vi "ABB Norma 5000 panel.vi"() -> ()   [LabVIEW 2017]
uses:
  ABB global.vi
panel:
  out "Total":T1
  out "norma 5000 parms out":T2
  out "L 3":T1
  out "L 2":T1
  out "L1":T1
  in  "Exit":bool
  # "NORMA 5000 Power Analyzer"
  # "Norma 5000 Power Analyzer"
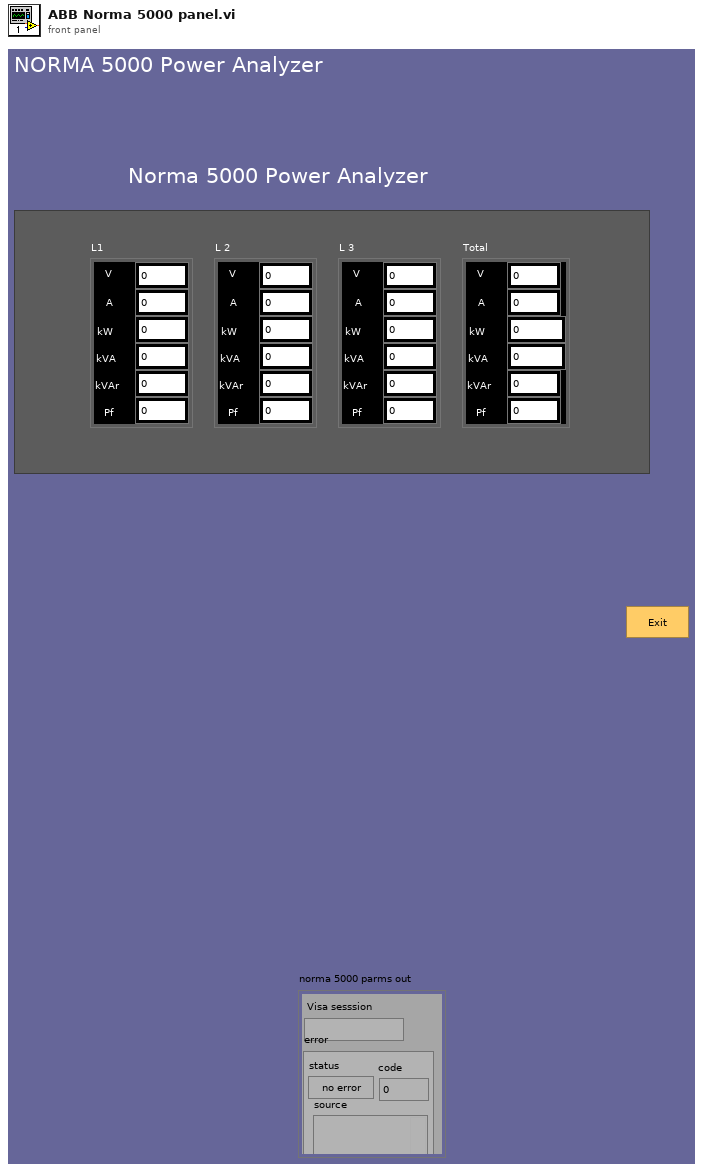
[diagram p1: front panel]
types:
  T1 = cluster{"V":dbl, "A":dbl, "kW":dbl, "kVA":dbl, "kVAr":dbl, "Pf":dbl}
  T2 = cluster{"Visa sesssion":refnum<visa-resource-name>, "error":errorcluster}
  T3 = cluster{"VT Primary":dbl, "VT Secondary":dbl, "CT  Primary":dbl, "CT Secondary":dbl, "Current Shunt":enum16{"Internal", "External"}, "Averaging interval":dbl}
  T4 = cluster{"Simulate Norma":bool, "Norma 5000 Address":u8, "WebDaq IP Address":string, "Simulate cDAQ":bool}
  T5 = cluster{"V":dbl, "A":dbl, "W":dbl, "VA":dbl, "VAr":dbl, "Pf":dbl}
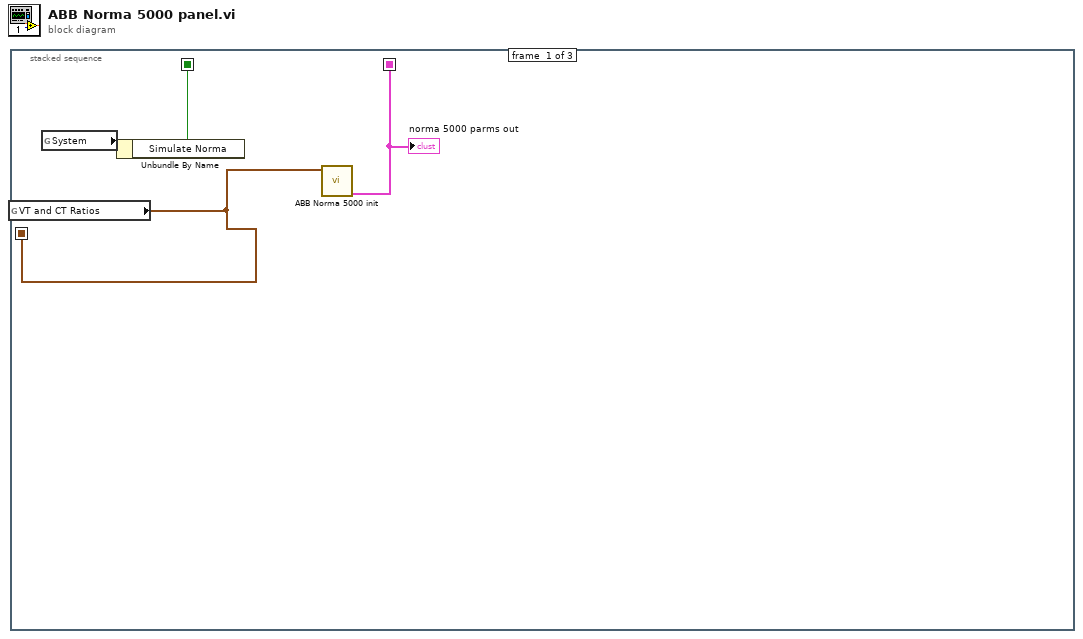
[diagram p0: block diagram]
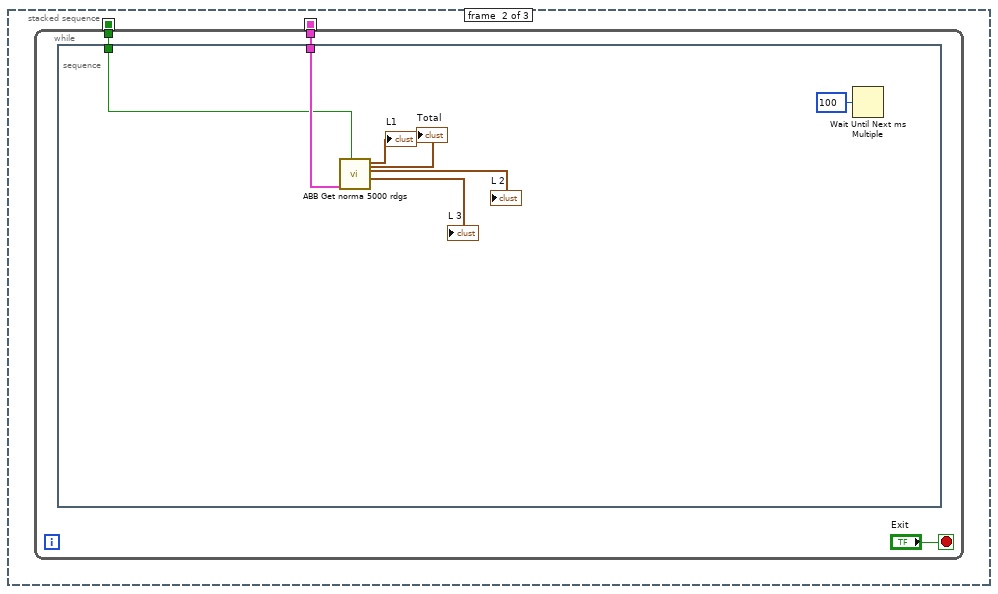
[diagram p2: hidden frame]
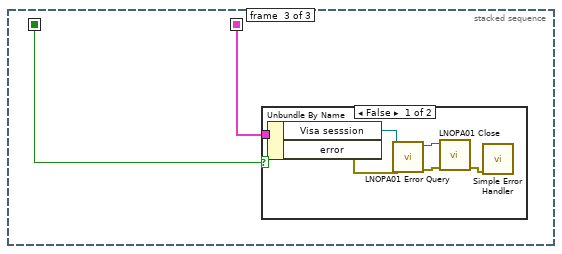
[diagram p3: hidden frame]
diagram:
  n1 = stacked-sequence {
    seq-local: [w4 _ _] -> [_ w6 w18]
    seq-local: [w2 _ _] -> [_ w5 w17]
    seq-local: [w1 _ _] -> [_ _ _]
    frame #0 {
      n2 = global read "ABB global.vi" "VT and CT Ratios"() -> (w1:T3)
      n3 = global read "ABB global.vi" "System"() -> (w3:T4)
      n4 = Unbundle By Name(w3) -> ("Simulate Norma"=w2:bool)
      n5 = call "ABB Norma 5000 init.vi"("VT and CT Ratios"=w1) -> ("norma 5000 parms out"=w4:T2)  [unwired: 10 in]
      "norma 5000 parms out" <- w4
    }
    frame #1 {
      n6 = while {
        tunnel: w6 -> [w8]
        tunnel: w5 -> [w7]
        stop <- "Exit" stop-if-true
        n7 = stacked-sequence {
          tunnel: w8 -> [w15]
          tunnel: w7 -> [w11]
          frame #0 {
            n8 = call "ABB Get norma 5000 rdgs.vi"("simulate"=w11, "norma 5000 parms in"=w15) -> ("L 3"=→"L 3":T5, "L 2"=→"L 2":T5, "L1"=→"L1":T5, "Total"=→"Total":T5)  [unwired: 5 in, 1 out]
            n9 = Wait Until Next ms Multiple(millisecond multiple=u32 100) -> ()  [unwired: 1 out]
          }
        }
      }
    }
    frame #2 {
      n10 = case shown="False" w17 {
        tunnel: w18 -> [w21 _]
        frame False {
          n11 = Unbundle By Name(w21) -> ("Visa sesssion"=w20:refnum<visa-resource-name>, "error"=w19:errorcluster)
          n12 = call "LNOPA01 Error Query.vi"("error in (no error)"=w19, "VISA session"=w20) -> ("error out"=w22:errorcluster, "dup VISA session"=w23:refnum<visa-resource-name>)  [unwired: 6 in, 2 out]
          n13 = call "LNOPA01 Close.vi"("error in (no error)"=w22, "VISA session"=w23) -> ("error out"=w24:errorcluster)  [unwired: 9 in]
          n14 = call <vilib>:"Simple Error Handler.vi"("error in (no error)"=w24) -> ()  [unwired: 4 in, 5 out]
        }
        frame True {
        }
      }
    }
  }
